vi "VI Store Launcher.vi"   [LabVIEW 2015]
uses:
  VI Store/VIStore Actor/VIStore.lvclass
  <vilib>/ActorFramework/Actor/Actor.lvclass
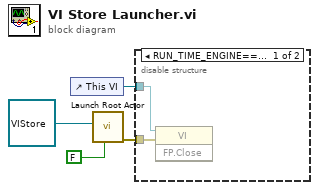
[diagram p0: block diagram]
diagram:
  n1 = control-ref of="This VI"() -> (w2:refnum<vi>)
  n2 = call <vilib>:"Launch Root Actor.vi"("Open Actor Core front panel? (F)"=FALSE, "Actor"=refnum<class "VIStore.lvclass"> refnum ("VI App Store.lvlib:VIStore.lvclass")) -> ("error out"=w1:errorcluster)  [unwired: 8 in, 1 out]
  n3 = disable-structure shown="RUN_TIME_ENGINE==True||Debug==False" {
    disable-tunnel: w2 -> [w6 _]
    disable-tunnel: w1 -> [w5 _]
    frame condition #0 {
      n4 = invoke class="VI" method="FP.Close"(reference=w6, error in=w5) -> ()  [unwired: 1 in, 3 out]
    }
    frame condition #1 (active) {
    }
  }
